vi "Setup UI.vi"(8 "error in (no error)":errorcluster, 10 "Set UI to input? (F)":bool, 11 "Lockin and Fluke Multimeter in":refnum<class "Lockin and Keithley Multimeter.lvclass">) -> (0 "error out":errorcluster, 3 "Lockin and Fluke Multimeter out":refnum<class "Lockin and Keithley Multimeter.lvclass">)   [LabVIEW 2023, in "Lockin and Keithley Multimeter.lvclass"]
doc: "Setup UI constructs an object -- populates its member fields -- from a front panel the user can see. The VI should be as simple as possible so that a UI loop can poll it continuously for updates. \n\nThe VI is designed to be used as a subPanel within another VI. Wire true to \"Set UI to input\" only on the first call, just after inserting this VI into a subPanel, to populate its controls with the class's current values.\n\nSetup UI is distinct from the class constructor. Class constructors are not polymorphic, yet configure dialogs need to configure objects without knowing their type -- and polymorphism is the necessary solution. Thus, Setup UI is a polymorphic class constructor. This continously polled \"Setup UI\" concept is a kludge: a better idea would be an XControl, but those require a steeper learning curve."
uses:
  Lockin and Keithley Multimeter.lvclass
  Lockin/Sensitivity.ctl
  Lockin and Keithley Multimeter.lvclass/Lockin and Keithley Multimeter.ctl
  Utility Classes/Readable/Readable.lvclass
  Lockin/sr830/SR830.lvlib
  Lockin/Lockin SR830.lvclass
panel:
  in  "Experiment":enum16{"CD", "EA", "None"}(ring)=enum."None"
  in  "Keithley Multiplier":dbl=1.0
  in  "Keithley Values":T1={"range (auto:0)"=0, "range value (volts)"=1000.0, "resolution (4.5 digits:3)"=7, "integration time (0:auto)"=0, "integ. value"=0.01667, "digital filter (off:0)"=0, "advanced filter (off:0)"=0, "dig. filter count"=10.0, "reference (off:0)"=0, "reference value (volts)"=0.0, "noise tolerance (%)"=1.0} {"noise tolerance (%)" min=0.0 max=100.0 step=1.0 format="%^.2e"; "reference value (volts)" min=-1100.0 max=1100.0 format="%^.2e"; "reference (off:0)" items=["off", "set reference value"]; "dig. filter count" min=1.0 max=100.0 step=1.0 format="%^.2e"; "advanced filter (off:0)" items=["off", "enabled"]; "digital filter (off:0)" items=["off", "auto filter", "auto filter once", "moving filter", "repeating filter"]; "integ. value" format="%^.2e"; "integration time (0:auto)" items=["automatic", "automatic once", "set to minimum", "set to maximum", "set aperature value", "set NPLC value"]; "resolution (4.5 digits:3)" items=["auto resolution", "auto resolution once", "3.5 digits", "4.5 digits", "5.5 digits", "6.5 digits", "7.5 digits", "8.5 digits"]; "range (auto:0)" items=["autorange", "autorange once", "set min range", "set max range", "set range value"]; "range value (volts)" min=0.2 max=1000.0 format="%^.2e"}
  in  "Keithley Offset":dbl
  in  "Set Properties":bool
  in  "Tau":u16(ring) items=["10 us", "30 us", "100 us", "300 us", "1 ms", "3 ms", "10 ms", "30 ms", "100 ms", "300 ms", "1 s", "3 s", "10 s", "30 s", "100 s", "300 s", "1 ks", "3 ks", "10 ks", "30 ks"]
  in  "Sensitivity":T2 items=["2 nV", "5 nV", "10 nV", "20 nV", "50 nV", "100 nV", "200 nV", "500 nV", "1 uV", "2 uV", "5 uV", "10 uV", "20 uV", "50 uV", "100 uV", "200 uV", "500 uV", "1 mV", "2 mV", "5 mV", "10 mV", "20 mV", "50 mV", "100 mV", "200 mV", "500 mV", "1 V"]
  out "Reference mode":enum16{"external", "internal"}(ring)
  out "Frequency":dbl[unit]
  # "Lockin & Keithley Reader Setup"
  # "SR830"
  # "Keithley Multimeter"
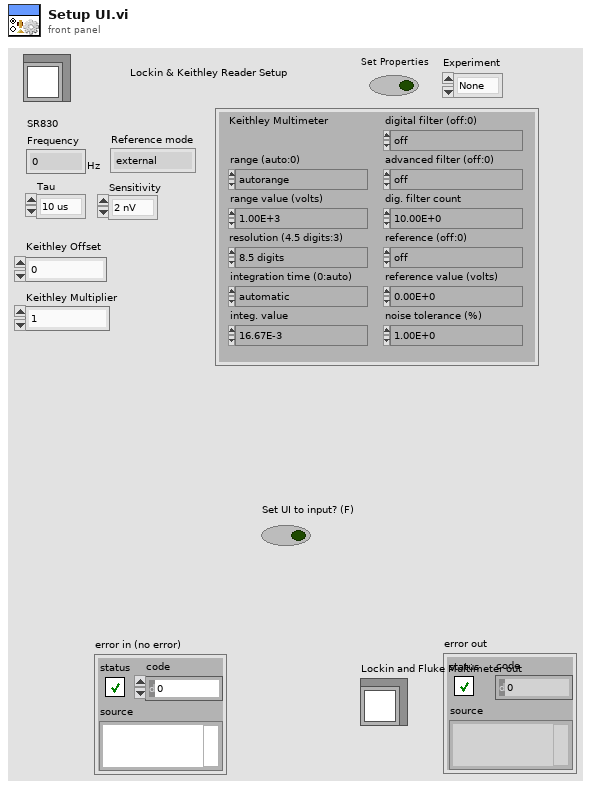
[diagram p1: front panel]
types:
  T1 = cluster{"range (auto:0)":u16, "range value (volts)":dbl, "resolution (4.5 digits:3)":u16, "integration time (0:auto)":u16, "integ. value":dbl, "digital filter (off:0)":u16, "advanced filter (off:0)":u16, "dig. filter count":dbl, "reference (off:0)":u16, "reference value (volts)":dbl, "noise tolerance (%)":dbl}
  T2 = typedef "Lockin SR830.lvclass/Sensitivity.ctl" = u16
  T3 = typedef "SR830.lvlib/Tau.ctl" = u16
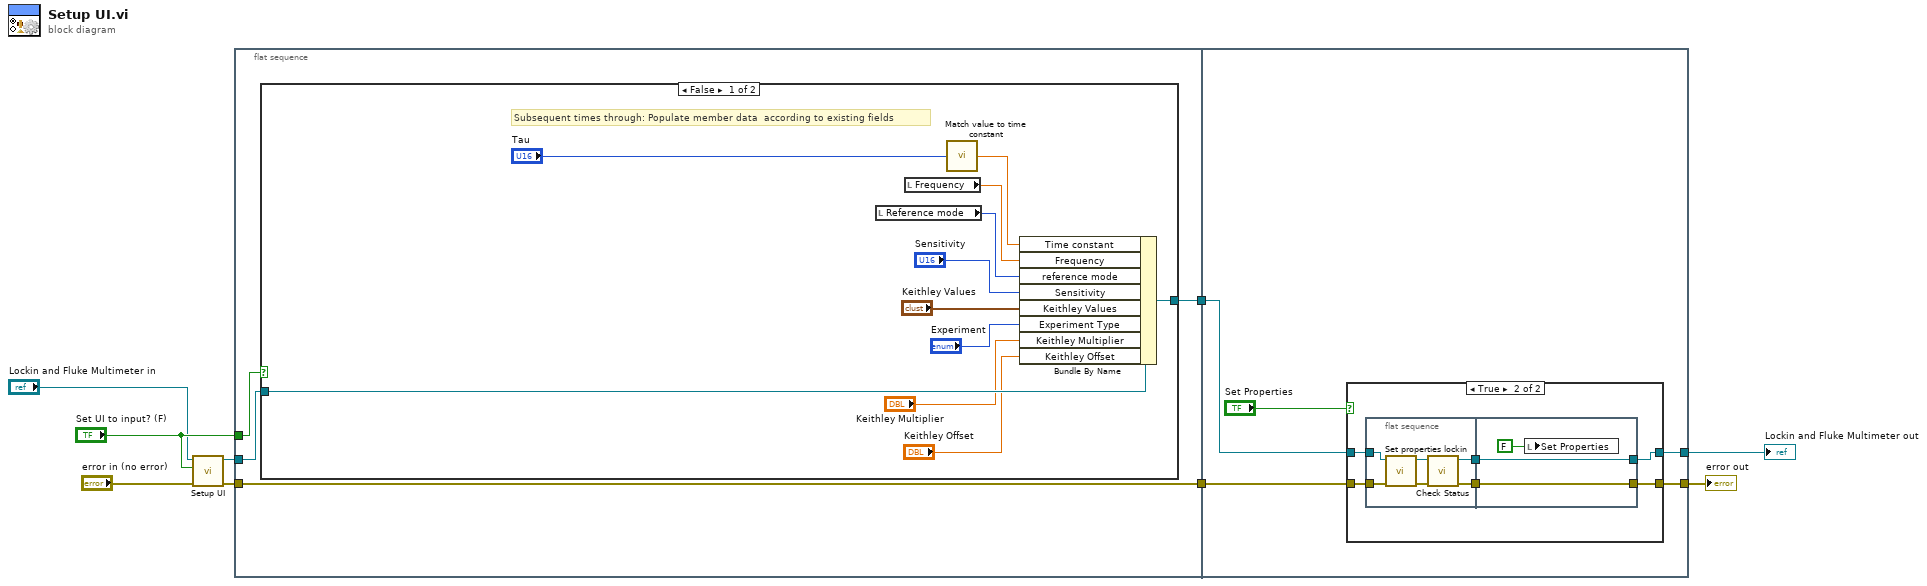
[diagram p0: block diagram]
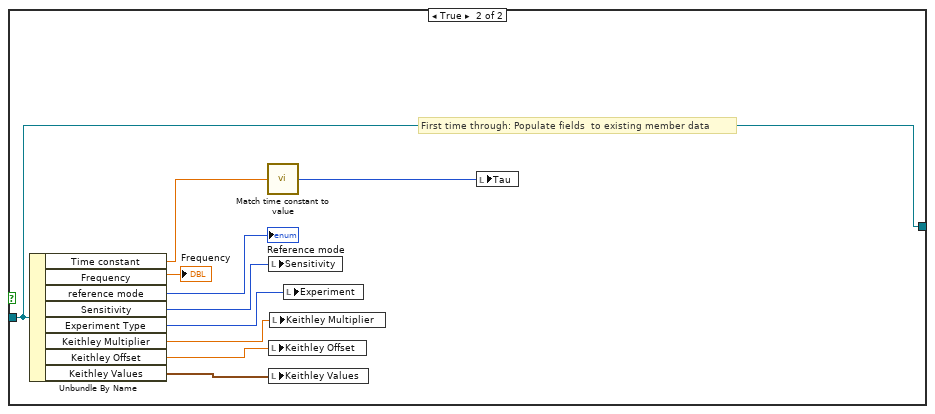
[diagram p2: hidden frame]
diagram:
  n1 = call-parent "Setup UI.vi"("error in (no error)"="error in (no error)", "Set UI to input? (F)"="Set UI to input? (F)", "Instrument in"="Lockin and Fluke Multimeter in") -> ("error out"=w4:errorcluster, "Instrument out"=w7:refnum<class "Lockin and Keithley Multimeter.lvclass">)  [unwired: 7 in]
  n2 = flat-sequence {
    tunnel: "Set UI to input? (F)" -> [w13]
    tunnel: w7 -> [w12]
    tunnel: [w11] -> w6
    tunnel: [w10] -> w5
    tunnel: w4 -> [w10]
    tunnel: w6 -> [w37]
    tunnel: w5 -> [w38]
    tunnel: [w36] -> w3
    tunnel: [w35] -> w2
    frame #0 {
      n3 = case shown="False" w13 {
        tunnel: w12 -> [w24 w31]
        tunnel: [w20 w31] -> w11
        frame False {
          # "Subsequent times through: Populate member data  according to existing fields"
          n4 = local read "Reference mode"() -> (w19:enum16{"external", "internal"})
          n5 = local read "Frequency"() -> (w18:dbl[unit])
          n6 = call "Match value to time constant.vi"("Tau"="Tau") -> ("time constant"=w22:dbl[unit])
          n7 = Bundle By Name(cluster=w24, "Time constant"=w22, "Frequency"=w18, "reference mode"=w19, "Sensitivity"="Sensitivity", "Keithley Values"="Keithley Values", "Experiment Type"="Experiment", "Keithley Multiplier"="Keithley Multiplier", "Keithley Offset"="Keithley Offset") -> (w20:refnum<class "Lockin and Keithley Multimeter.lvclass">)
        }
        frame True {
          # "First time through: Populate fields  to existing member data"
          n8 = Unbundle By Name(w31) -> ("Time constant"=w34:dbl[unit], "Frequency"=→"Frequency":dbl[unit], "reference mode"=→"Reference mode":enum16{"external", "internal"}, "Sensitivity"=w32:T2, "Experiment Type"=w26:enum16{"CD", "EA", "None"}, "Keithley Multiplier"=w25:dbl, "Keithley Offset"=w28:dbl, "Keithley Values"=w27:T1)
          n9 = call "Match time constant to value.vi"("Time constant"=w34) -> ("Tau"=w33:T3)
          n10 = local write "Sensitivity"(w32) -> ()
          n11 = local write "Keithley Offset"(w28) -> ()
          n12 = local write "Keithley Values"(w27) -> ()
          n13 = local write "Keithley Multiplier"(w25) -> ()
          n14 = local write "Experiment"(w26) -> ()
          n15 = local write "Tau"(w33) -> ()
        }
      }
    }
    frame #1 {
      n16 = case shown="True" "Set Properties" {
        tunnel: w38 -> [w40 w47]
        tunnel: w37 -> [w41 w46]
        tunnel: [w41 w44] -> w36
        tunnel: [w40 w43] -> w35
        frame False {
        }
        frame True {
          n17 = flat-sequence {
            tunnel: w47 -> [w51]
            tunnel: w46 -> [w50]
            tunnel: [w49] -> w45
            tunnel: [w48] -> w42
            tunnel: w45 -> [w55]
            tunnel: [w55] -> w44
            tunnel: [w54] -> w43
            tunnel: w42 -> [w54]
            frame #0 {
              n18 = call "Set properties lockin.vi"("error in (no error)"=w51, "Lockin and Keithley Multimeter in"=w50) -> ("error out"=w52:errorcluster, "Lockin and Keithley Multimeter out"=w53:refnum<class "Lockin and Keithley Multimeter.lvclass">)  [unwired: 8 in]
              n19 = call-dynamic "Check Status.vi"("error in (no error)"=w52, "Lockin and Keithley Multimeter in"=w53) -> ("error out"=w48:errorcluster, "Lockin and Keithley Multimeter out"=w49:refnum<class "Lockin and Keithley Multimeter.lvclass">)  [unwired: 6 in, 2 out]
            }
            frame #1 {
              n20 = local write "Set Properties"(FALSE ("Set Parameters")) -> ()
            }
          }
        }
      }
    }
  }
  "error out" <- w2
  "Lockin and Fluke Multimeter out" <- w3
